vi "日期字符串格式至时间格式转换(子VI).vi"(11 "data[0]":string) -> (3 "time stamp":timestamp format="%<%Y/%m/%d %H:%M:%S>T")   [LabVIEW 2016]
uses:
  <vilib>/Utility/miscctls.llb/LVDateTimeRec.ctl
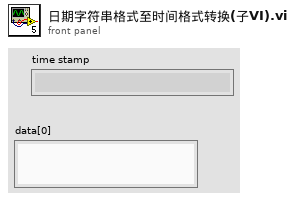
[diagram p1: front panel]
types:
  T1 = typedef "LVDateTimeRec.ctl" = cluster{"fractional second":dbl, "second":i32, "minute":i32, "hour":i32, "day of month":i32, "month":i32, "year":i32, "day of week":i32, "day of year":i32, "DST":i32}
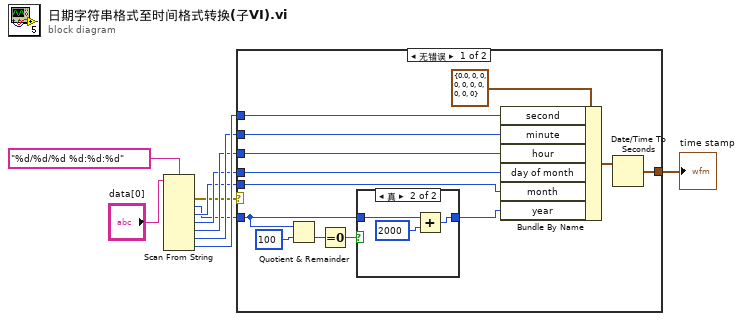
[diagram p0: block diagram]
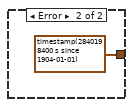
[diagram p3: hidden frame]
diagram:
  n1 = Scan From String(format string="%d/%d/%d %d:%d:%d" ("格式字符串"), input string="data[0]") -> (error out=w2:errorcluster, output 1=w5:i32, output 2=w6:i32, output 3=w7:i32, output 4=w8:i32, output 5=w9:i32, output 6=w10:i32)  [unwired: 8 in, 2 out]
  n2 = case shown="无错误" w2 {
    tunnel: w10 -> [w22 _]
    tunnel: w9 -> [w21 _]
    tunnel: w8 -> [w20 _]
    tunnel: w7 -> [w19 _]
    tunnel: w6 -> [w18 _]
    tunnel: w5 -> [w14 _]
    tunnel: [w16 timestamp(2840198400 s since 1904-01-01) ("time stamp")] -> w1
    frame No Error {
      n3 = Quotient & Remainder(x=w14, y=100) -> (floor(x/y)=w13:i32)  [unwired: 1 out]
      n4 = Equal To 0?(x=w13) -> (x = 0?=w12:bool)
      n5 = case shown="真" w12 {
        tunnel: w14 -> [w24 w27]
        tunnel: [w24 w25] -> w11
        frame False {
        }
        frame True {
          n6 = Add(x=w27, y=2000) -> (x+y=w25:i32)
        }
      }
      n7 = Bundle By Name(cluster=T1 {"fractional second"=0.0, "second"=0, "minute"=0, "hour"=0, "day of month"=0, "month"=0, "year"=0, "day of week"=0, "day of year"=0, "DST"=0} ("日期时间记录"), "second"=w22, "minute"=w21, "hour"=w20, "day of month"=w19, "month"=w18, "year"=w11) -> (w23:T1)
      n8 = Date/Time To Seconds(2:w23) -> (0:w16:timestamp)  [unwired: 1 in]
    }
    frame Error {
    }
  }
  "time stamp" <- w1
